vi "Map Type.vi"(8 "error in (no error)":errorcluster, 10 "Type":variant, 11 "Database Manager in":refnum<class "Database Manager.lvclass">) -> (0 "error out":errorcluster, 1 "Mapped Type":string, 3 "Database Manager out":refnum<class "Database Manager.lvclass">)   [LabVIEW 2019, in "HierDAL Library.lvlib" / "Database.lvlib" / "Database Manager.lvclass"]
doc: "Maps a G type to its corresponding database type using a provided mapping.\n\n<b>Type</b> - The G type to map to a database type (e.g., I32, DBL).\n<b>Mapped Type</b> - The corresponding database type as a string."
uses:
  Database Manager.lvclass
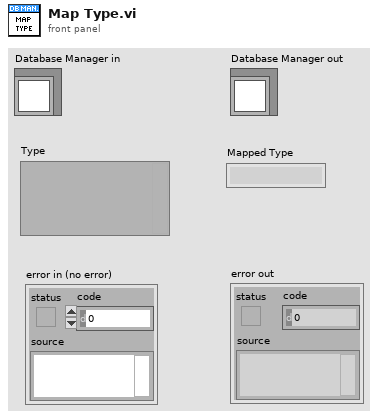
[diagram p1: front panel]
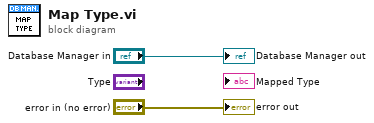
[diagram p0: block diagram]
diagram:
  "error out" <- "error in (no error)"
  "Database Manager out" <- "Database Manager in"
